vi "Initialize EXCEL.vi"(8 "error in (no error)":errorcluster, 11 "NI_report in":refnum<class "NI_report.lvclass">) -> (0 "error out":errorcluster, 3 "NI_report out":refnum<class "NI_report.lvclass">)   [LabVIEW 2016, in "Report.lvlib"]
uses:
  Report.lvlib
  <vilib>/Utility/NIReport.llb/NI_report.lvclass
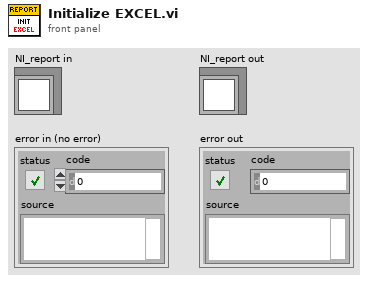
[diagram p1: front panel]
types:
  T1 = cluster{"Charset (-1)":i16, "Weight (-1)":i16, "Name":string, "Size":string}
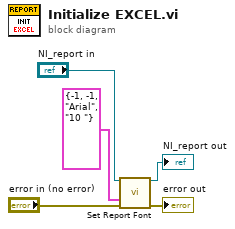
[diagram p0: block diagram]
diagram:
  n1 = call-dynamic "Set Report Font.vi"("report in"="NI_report in", "font settings"=T1 {"Charset (-1)"=-1, "Weight (-1)"=-1, "Name"="Arial", "Size"="10 "}, "error in (no error)"="error in (no error)") -> ("report out"=→"NI_report out":refnum<class "NI_report.lvclass">, "error out"=→"error out":errorcluster)  [unwired: 10 in, 1 out]
